vi "Sequence.Start.vi"(8 "error in":errorcluster, 10 "UserSets":T11, 11 "Data in":T1={"BeginTS"=timestamp(0 s since 1904-01-01), "EndTS"=timestamp(0 s since 1904-01-01), "State"=enum."Init", "Status.Work"=enum."-", "Status.Process"=enum."-", "Status.Home"=enum."-", "Status.Wabco"=enum."-", "Status.Client"=enum."-", "BreakReason"=enum."-", "BreakSource"=enum."-", "DoorLock"=FALSE, "Status.Prod"=[], "UserAction"={"Stop"=FALSE, "Pause"=FALSE, "Next"=FALSE}, "UserData"={"GuiMode"=enum."Process", "Test"={"IgnoreResults"=FALSE, "IgnoreImages"=FALSE, "ServiceMode"=FALSE}, "ContinueOrder"=FALSE}, "Error"={"status"=FALSE, "code"=0, "source"=""}, "Code"={"Ready"=FALSE, "DoubleOrder"=FALSE, "OrderDone"=FALSE, "AllowSingleSlot"=FALSE, "CheckDM"=FALSE, "ThresholdA"=0, "ThresholdB"=0, "Plate"=enum."Wabco", "ImgPath"=path "", "Variant"={"State"=enum."Init", "ImgPath"=path "", "WabcoPlate"="", "WabcoProduct"="", "ClientProduct"="", "ClientPlate"="", "TotalQuantity"=0, "OrderQuantity"=0, "Serial"=0, "Wabco"={"LaserJob"="", "AdditionalTxt"="037", "FactoryCode"="", "RevID"=0, "ForkID"=0, "FailuresLimit"=0, "GlobalCnt"=0, "Bank"=0, "SerialFormat"=enum."6 dig", "CoordA"={"X"=0.0, "Y"=0.0, "Angle"=0.0}, "CoordB"={"X"=0.0, "Y"=0.0, "Angle"=0.0}, "DMCconfig"=0}, "Client"={"LaserJob"="", "AdditionalTxt"="", "FactoryCode"="037", "RevID"=0, "ForkID"=0, "FailuresLimit"=0, "GlobalCnt"=0, "Bank"=0, "SerialFormat"=enum."6 dig", "CoordA"={"X"=0.0, "Y"=0.0, "Angle"=0.0}, "CoordB"={"X"=0.0, "Y"=0.0, "Angle"=0.0}, "DMCconfig"=0}}}, "Rotations"=0, "ProdIdx"=0, "ProdDone"=[], "PrintedSerials-Wabco"=[], "PrintedSerials-Client"=[], "Counters-Wabco"={"Expected"=0, "Done"=0, "OK"=0, "NOK"=0, "NOKlimit"=0, "Part"=0, "PartOK"=0}, "Counters-Client"={"Expected"=0, "Done"=0, "OK"=0, "NOK"=0, "NOKlimit"=0, "Part"=0, "PartOK"=0}}) -> (0 "error out":errorcluster, 3 "Data out":T1={"BeginTS"=timestamp(0 s since 1904-01-01), "EndTS"=timestamp(0 s since 1904-01-01), "State"=enum."Init", "Status.Work"=enum."-", "Status.Process"=enum."-", "Status.Home"=enum."-", "Status.Wabco"=enum."-", "Status.Client"=enum."-", "BreakReason"=enum."-", "BreakSource"=enum."-", "DoorLock"=FALSE, "Status.Prod"=[], "UserAction"={"Stop"=FALSE, "Pause"=FALSE, "Next"=FALSE}, "UserData"={"GuiMode"=enum."Process", "Test"={"IgnoreResults"=FALSE, "IgnoreImages"=FALSE, "ServiceMode"=FALSE}, "ContinueOrder"=FALSE}, "Error"={"status"=FALSE, "code"=0, "source"=""}, "Code"={"Ready"=FALSE, "DoubleOrder"=FALSE, "OrderDone"=FALSE, "AllowSingleSlot"=FALSE, "CheckDM"=FALSE, "ThresholdA"=0, "ThresholdB"=0, "Plate"=enum."Wabco", "ImgPath"=path "", "Variant"={"State"=enum."Init", "ImgPath"=path "", "WabcoPlate"="", "WabcoProduct"="", "ClientProduct"="", "ClientPlate"="", "TotalQuantity"=0, "OrderQuantity"=0, "Serial"=0, "Wabco"={"LaserJob"="", "AdditionalTxt"="037", "FactoryCode"="", "RevID"=0, "ForkID"=0, "FailuresLimit"=0, "GlobalCnt"=0, "Bank"=0, "SerialFormat"=enum."6 dig", "CoordA"={"X"=0.0, "Y"=0.0, "Angle"=0.0}, "CoordB"={"X"=0.0, "Y"=0.0, "Angle"=0.0}, "DMCconfig"=0}, "Client"={"LaserJob"="", "AdditionalTxt"="", "FactoryCode"="037", "RevID"=0, "ForkID"=0, "FailuresLimit"=0, "GlobalCnt"=0, "Bank"=0, "SerialFormat"=enum."6 dig", "CoordA"={"X"=0.0, "Y"=0.0, "Angle"=0.0}, "CoordB"={"X"=0.0, "Y"=0.0, "Angle"=0.0}, "DMCconfig"=0}}}, "Rotations"=0, "ProdIdx"=0, "ProdDone"=[], "PrintedSerials-Wabco"=[], "PrintedSerials-Client"=[], "Counters-Wabco"={"Expected"=0, "Done"=0, "OK"=0, "NOK"=0, "NOKlimit"=0, "Part"=0, "PartOK"=0}, "Counters-Client"={"Expected"=0, "Done"=0, "OK"=0, "NOK"=0, "NOKlimit"=0, "Part"=0, "PartOK"=0}})   [LabVIEW 2016]
uses:
  Sequence.UserData.ctl
  Sequence.MainMode.ctl
  Gui/MainGui.TestOptions.ctl
  Sequence.Data.ctl
  Sequence.State.ctl
  Sequence.Step.Status.ctl
  Sequence.Test.BreakReason.ctl
  Sequence.Test.BreakSource.ctl
  Sequence.Test.Status.ctl
  Sequence.Slot.StatusData.ctl
  Sequence.Test.Unload.Status.ctl
  Sequence.Prod.StatusData.ctl
  Sequence.UserActions.ctl
  Sequence.Code.Sets.ctl
  Sequence.PlateType.ctl
  Logger/Logger.Variant.Sets.ctl
  Station/Station.Changeover.State.vi
  Station/Station.Plate.Properties.ctl
  Sequence.Code.SerialFormat.ctl
  Drivers/V7310/LowLevel/V7310.Job.Sets.ctl
  Sequence.Counters.ctl
  tools/EventLog/EventLog.EventSource.ctl
  Sequence.SerialsFglb.Action.ctl
  Sequence.SerialsFglb.SerialData.ctl
  Station/Station.ProductSlot.ctl
  tools/Translator/Translator.Message.ctl
  Station/Station.Global.vi
  tools/EventLog/EventLog.New(array).vi
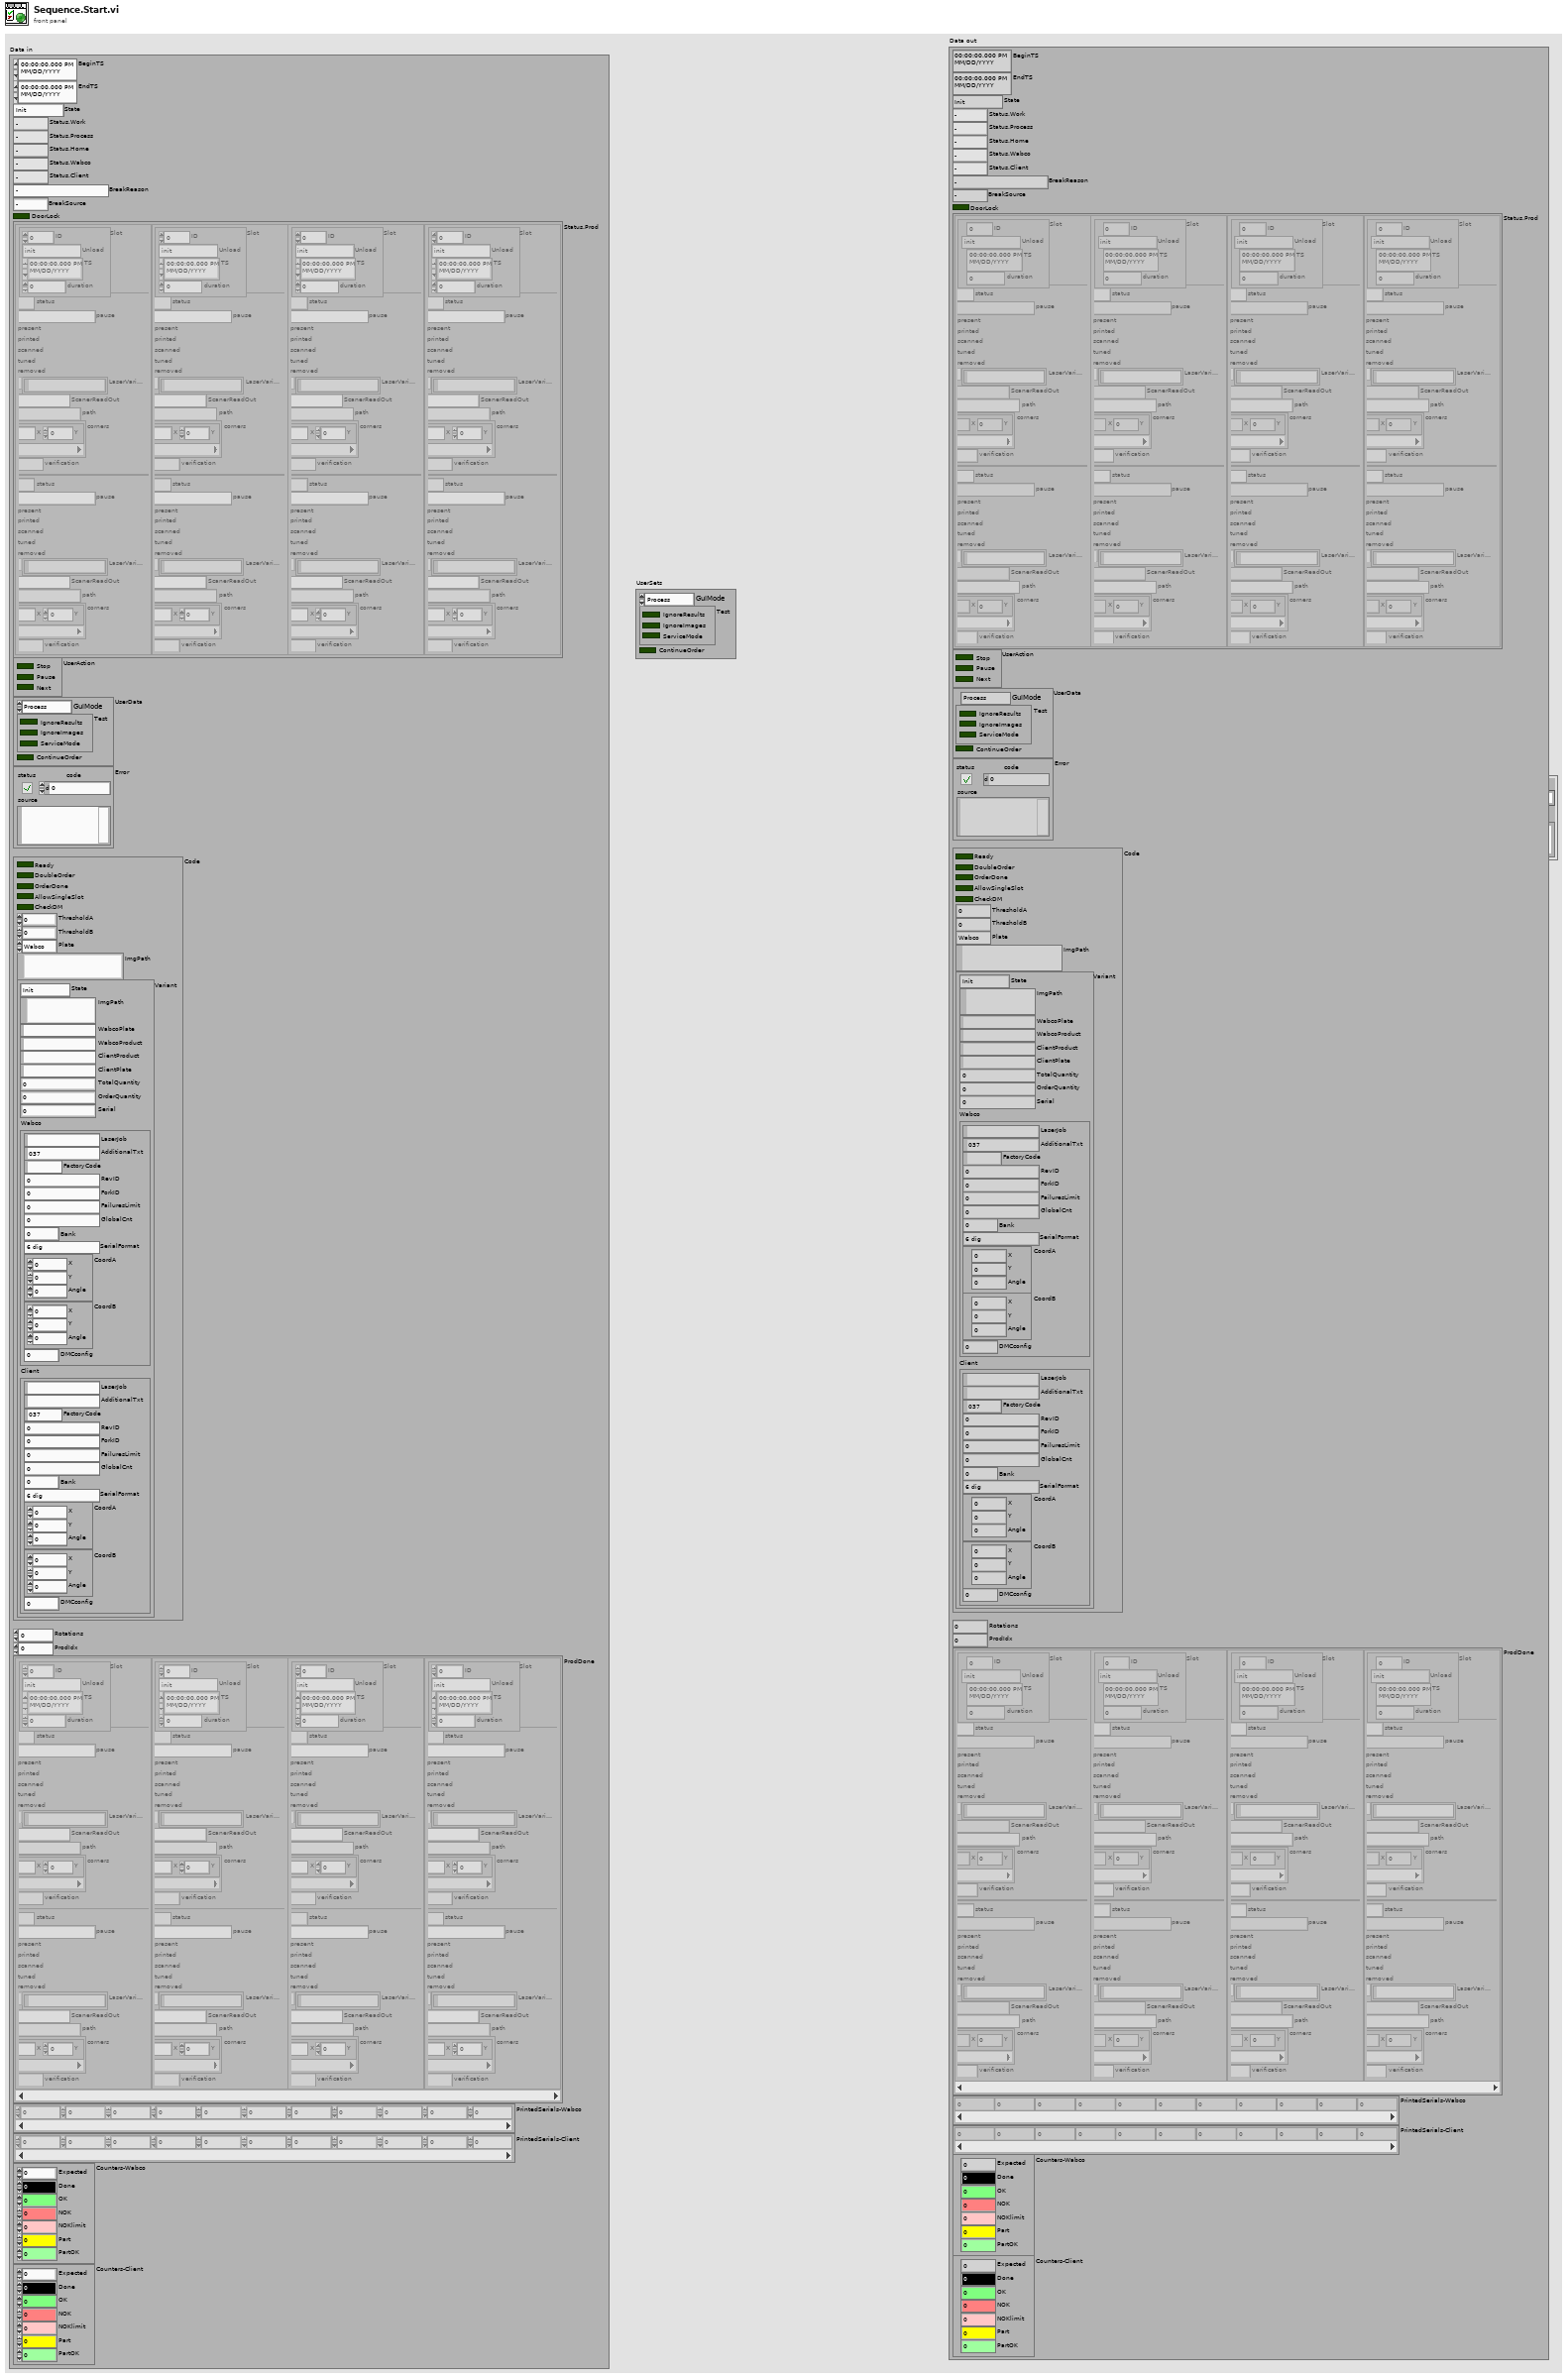
[diagram p1: front panel]
types:
  T1 = typedef "Sequence.Data.ctl" = cluster{"BeginTS":timestamp, "EndTS":timestamp, "State":T2, "Status.Work":T3, "Status.Process":T3, "Status.Home":T3, "Status.Wabco":T3, "Status.Client":T3, "BreakReason":T4, "BreakSource":T5, "DoorLock":bool, "Status.Prod":T6[], "UserAction":T10, "UserData":T11, "Error":errorcluster, "Code":T14, "Rotations":i32, "ProdIdx":i32, "ProdDone":T6[], "PrintedSerials-Wabco":i32[], "PrintedSerials-Client":i32[], "Counters-Wabco":T21, "Counters-Client":T21}
  T2 = typedef "Sequence.State.ctl" = enum16{"Init", "Idle", "Home", "Work", "Run", "Pause"}
  T3 = typedef "Sequence.Step.Status.ctl" = enum16{"-", "Pending", "Running", "Skipped", "Passed", "Failed", "Done", "Error", "Aborted", "Stopped"}
  T4 = typedef "Sequence.Test.BreakReason.ctl" = enum16{"-", "NOK container", "OK container", "Rev empty", "Rev missing", "Rev wrong", "Fork missing", "Fork wrong", "NOK limit", "Unload failure", "Single slot", "Part done", "Err: Prod move work", "Err: Prod move home", "Err: Prod lift work", "Err: Prod lift home", "Err: Prod Arm Work", "Err: Prod Arm NOK", "Err: Prod Arm OK", "Err: Prod NOK suck", "Err: Prod NOK drop", "Err: Prod OK missing", "Err: Prod OK suck", "Err: Prod OK drop"}
  T5 = typedef "Sequence.Test.BreakSource.ctl" = enum16{"-", "A", "B", "A/B"}
  T6 = typedef "Sequence.Test.Status.ctl" = cluster{"Slot":T7, "A":T9, "B":T9}
  T7 = typedef "Sequence.Slot.StatusData.ctl" = cluster{"ID":i32, "Unload":T8, "TS":timestamp, "duration":u32}
  T8 = typedef "Sequence.Test.Unload.Status.ctl" = enum16{"init", "check NOK", "check OK", "wait on NOK", "wait on OK", "wait on Unload", "done"}
  T9 = typedef "Sequence.Prod.StatusData.ctl" = cluster{"status":T3, "pause":T4, "present":bool, "printed":bool, "scanned":bool, "tuned":bool, "removed":bool, "LaserVariables":string[], "ScanerReadOut":string, "path":path, "corners":cluster{"X":i32, "Y":i32}[], "verification":u8}
  T10 = typedef "Sequence.UserActions.ctl" = cluster{"Stop":bool, "Pause":bool, "Next":bool}
  T11 = typedef "Sequence.UserData.ctl" = cluster{"GuiMode":T12, "Test":T13, "ContinueOrder":bool}
  T12 = typedef "Sequence.MainMode.ctl" = enum16{"Process", "Base", "Order", "Manual", "Logs", "Results", "Stats", "DMC Config"}
  T13 = typedef "MainGui.TestOptions.ctl" = cluster{"IgnoreResults":bool, "IgnoreImages":bool, "ServiceMode":bool}
  T14 = typedef "Sequence.Code.Sets.ctl" = cluster{"Ready":bool, "DoubleOrder":bool, "OrderDone":bool, "AllowSingleSlot":bool, "CheckDM":bool, "ThresholdA":u8, "ThresholdB":u8, "Plate":T15, "ImgPath":path, "Variant":T16}
  T15 = typedef "Sequence.PlateType.ctl" = enum16{"Wabco", "Client"}
  T16 = typedef "Logger.Variant.Sets.ctl" = cluster{"State":T17, "ImgPath":path, "WabcoPlate":string, "WabcoProduct":string, "ClientProduct":string, "ClientPlate":string, "TotalQuantity":u16, "OrderQuantity":u16, "Serial":i32, "Wabco":T18, "Client":T18}
  T17 = typedef "Station.Changeover.State.vi" = enum16{"Init", "Scaning", "NOK", "Wait for ack", "Ready"}
  T18 = typedef "Station.Plate.Properties.ctl" = cluster{"LaserJob":string, "AdditionalTxt":string, "FactoryCode":string, "RevID":u8, "ForkID":u8, "FailuresLimit":u16, "GlobalCnt":i32, "Bank":u8, "SerialFormat":T19, "CoordA":T20, "CoordB":T20, "DMCconfig":i32}
  T19 = typedef "Sequence.Code.SerialFormat.ctl" = enum8{"", "6 dig", "7 dig"}
  T20 = typedef "V7310.Job.Sets.ctl" = cluster{"X":dbl, "Y":dbl, "Angle":dbl}
  T21 = typedef "Sequence.Counters.ctl" = cluster{"Expected":u16, "Done":u16, "OK":u16, "NOK":u16, "NOKlimit":u16, "Part":u16, "PartOK":u16}
  T22 = typedef "Translator.Message.ctl" = enum16{"-", "Event confirmed", "Log out", "Log in", "Shutdown", "Cancel", "Start", "Begin time", "End time", "Duration", "Service Mode", "Ignore Results", "Serial Format", "On", "Off", "OK", "NOK", "NOK %s", "Home", "Work", "Close", "Open", "In progress...", "Missing", "Empty", "Hardware failure", "Initial", "Default", "Total", "Out of range", "Free disk space is below 1GB - contact technician", "Error %d >> %s", "Error %d >> %s >> %s", "Msg %d >> %s", "Laser msg %d %s", "Laser cmd error %s %d", "Laser cmd failed %s", "Laser cmd warning %s", "Laser disconnected", "Laser status %s", "Laser already started", "Laser job unkonwn %s", "Laser job missing %s", "Laser job select failure %s", "Unable to start laser printing (%s)", "Unable to stop laser printing (%s)", "Laser marking aborted", "Laser marking timeout", "Unable to reset Laser Interlock (%s)", "Unable to trigger Laser. Laser not ready (%s)", "Laser job '%s' coordinates not configured", "Starting %s", "Quitting %s", "Configured", "Initializing", "Quitting", "Loading", "Loaded %d results", "Loaded %d events", "Running", "Stopped", "Summary", "Laser", "Do you want to continue?", "Do you want to delete the configuration?", "The configuration is being used by an order. Unable to delete!", "Press confirm button", "Station is not based. Do you want to exit?", "Station requires changeover. Do you want to run the test?", "Test options are not set as default. Do you want to continue?", "Formatting of WabcoNo is disabled. Do you want to continue?", "Product not detected. Do you want to continue?", "Product scan failed. Do you want to continue?", "Calibration", "Log out?", "System", "All", "IDLE", "Translating...%s", "Not found", "Alarm %s", "Run", "Skip", "Abort", "Repeat", "Please wait...", "Database disconnected", "Database disconnected - changeover disabled!", "Login to database successful", "Login to database failed: %d; %s", "Unable to check the product status of reference %d - database disconnected", "Unable to set the product status of reference %d - database disconnected", "Variant file backup %s", "Read variant (%s)", "Result", "Station armed!", "Station requires changeover!", "Select reference number...", "EMERGENCY BUTTON - press Control button", "EMERGENCY DOOR - press Control button", "Resetting Emergency...", "Unable to reset safety circuit - Emergency Button pressed", "Unable to reset safety circuit - Emergency Side Door open", "Station not based", "Station based", "Station not empty", "Station basing...", "No order", "Press Start to begin new order", "Scanning new order", "Order NOK. Correct or scan again", "Order OK. Press Accept", "Order ready", "Revolver incorrect", "Fork incorrect", "Revolver missing", "Revolver empty", "Container missing", "Offline results", "Offline statistics", "Updating statistics %.1f %%", "DMC Configurator", "Door open", "Close the front door", "Press start button", "Done. Open the front door", "Running...", "Running...%.1f %%", "Pause %s", "Pause %s. NOK container missing", "Pause %s. OK container missing", "Pause %s. Revolver empty", "Pause %s. Revolver missing", "Pause %s. Revolver incorrect", "Pause %s. Fork missing", "Pause %s. Fork incorrect", "Pause %s. Too many failures", "Pause %s. Unloading failure", "Pause %s. One slot is not working", "Pause %s. Part order is done. Empty OK container", "Pause %s. Unable to move product to slot", "Pause %s. Unable to move back product pusher", "Pause %s. Unable to lift product", "Pause %s. Unable to move back product lifter", "Pause %s. Unable to move product arm to Work", "Pause %s. Unable to move product arm to NOK", "Pause %s. Unable to move product arm to OK", "Pause %s. Unable to unsuck the NOK product", "Pause %s. Unable to drop the NOK product", "Pause %s. Product OK missing", "Pause %s. Unable to unsuck the OK product", "Pause %s. Unable to drop the OK product", "Stopping...", "File '%s' is missing", "File '%s' is broken", "File '%s' is running", "Log file started (%s)", "Log file ended (%s)", "Log file stopped (%s)", "Log file ignored (%s)", "Log file exported (%s)", "Log file export failed (%s)", "Wrong serial number in log file", "Wrong reference number in log file", "Test steps are missing", "%s = %.3f", "Process param '%s' not found in DB", "Process param '%s' wrong order", "Process param '%s' value %.3f out of limits (%.3f; %.3f)", "Step%d param '%s' not found in DB", "Step%d param '%s' wrong order", "Step%d param '%s' value %.3f out of limits (%.3f; %.3f)", "Step%d EV '%s' not found in DB", "Step%d EV '%s' wrong order", "\"%s\" not found in DB", "\"%s\" wrong order", "\"%s\" value %.3f out of limits (%.3f; %.3f)", "\"%s\" not found in software", "Process init (%s)", "Process started", "Process restarted", "Process run", "Process done", "Process done - remove OK container", "Process aborted", "Process aborted at work", "Process aborted at home", "Process error", "Process error at home", "Process error at work", "Process close", "Process pause", "Process continue", "Process door open", "Process door close", "Process pause at slot %s due to %s", "Select plate from the order to process", "Do you want to start the process?", "Do you want to continue the process?", "There is unfinished order. Do you want to put the new order?", "Product %s %d OK", "Product %s %d NOK", "Unable to unload the slot %s. Product missing in the slot", "Unable to unload the slot %s. Product already in the arm", "Unable to accept the product as OK. Product missing in slot %s", "Unable to accept the product as OK. Product could not drop into the container at slot %s", "Unable to accept the product as NOK. Product could not drop into the container at slot %s", "Scan failed. Error %s", "Scan failed. Scanner disconnected", "Scan failed. Wrong Wabco number %d, limit (%d,%d)", "Scan failed. Wrong serial number %d, limit (%d,%d)", "Scan failed. Wrong date %d, limit (%d,%d)", "Scan failed. Wrong product wabco number %d (expected %d)", "Scan failed. Wrong product serial number %d (expected > 0)", "Scan OK %s", "Scan failed. Unable to determine table position (%s)", "Scan failed. Timeout", "Tune failed. Scanner disconnected", "Tune failed. Timeout", "%s = %d", "%s = %d->%d", "Unable to set %s = %.2f - Air Pressure Inside off", "Unable to set digital output '%s' = %d", "Unable to activate air pressure inside - timeout", "Unable to activate air pressure inside - aborted", "Unable to switch on Air Main Valve - Air Pressure Inlet off", "Unable to switch on Air Main Valve - Door open", "Unable to switch off Air Main Valve - timeout", "Unable to switch off Air Main Valve - aborted", "Unable to rotate Table - timeout", "Unable to rotate Table - aborted", "Unable to rotate Table - Product Move not in Home position", "Unable to rotate Table - Air Pressure Inside off", "Unable to rotate Table - Product Lift A not in Home position", "Unable to rotate Table - Product Lift B not in Home position", "Unable to rotate Table - unlock before movement timeout", "Unable to rotate Table - lock after movement timeout", "Unable to move Table Lock to %s position - timeout", "Unable to move Table Lock to %s position - aborted", "Unable to move Table Lock to %s position - Air Pressure Inside off", "Unable to move Table Lock to %s position - Table not in position", "Unable to move Product Lift A to %s position - timeout", "Unable to move Product Lift B to %s position - timeout", "Unable to move Product Lift A to %s position - aborted", "Unable to move Product Lift B to %s position - aborted", "Unable to move Product Lift A to %s position - Air Pressure Inside off", "Unable to move Product Lift B to %s position - Air Pressure Inside off", "Unable to move Product Lift A to %s position - Table not locked", "Unable to move Product Lift B to %s position - Table not locked", "Unable to move Product Lift A to %s position - Product Arm not in Work position", "Unable to move Product Lift B to %s position - Product Arm not in Work position", "Unable to set Product Suction Gripper %s to %s - timeout", "Unable to set Product Suction Gripper %s to %s - aborted", "Unable to set Product Suction Gripper %s to %s - Air Pressure Inside off", "Unable to set Product Suction Gripper %s to %s - Table slot unkown", "Unable to move Product Arm to %s position - timeout", "Unable to move Product Arm to %s position - aborted", "Unable to move Product Arm to %s position - Air Pressure Inside off", "Unable to move Product Arm to %s position - Product Lift A not in Home position", "Unable to move Product Arm to %s position - Product Lift B not in Home position", "Unable to move Product to %s position - timeout", "Unable to move Product to %s position - aborted", "Unable to move Product to %s position - Air Pressure Inside off", "Unable to move Product to %s position - Table not in position"}
  T23 = typedef "Sequence.SerialsFglb.SerialData.ctl" = cluster{"TS":timestamp, "Slot":T24, "Serial":i32, "Global":bool}
  T24 = typedef "Station.ProductSlot.ctl" = enum8{"A", "B"}
  T25 = typedef "Sequence.SerialsFglb.Action.ctl" = enum16{"init", "get", "get next", "pass", "fail", "confirm", "clean"}
  T26 = typedef "EventLog.EventSource.ctl" = enum16{"All", "Gui", "Ref", "File", "Arch", "Seq", "CPX", "DB", "Laser", "Scan.P", "Scan.O"}
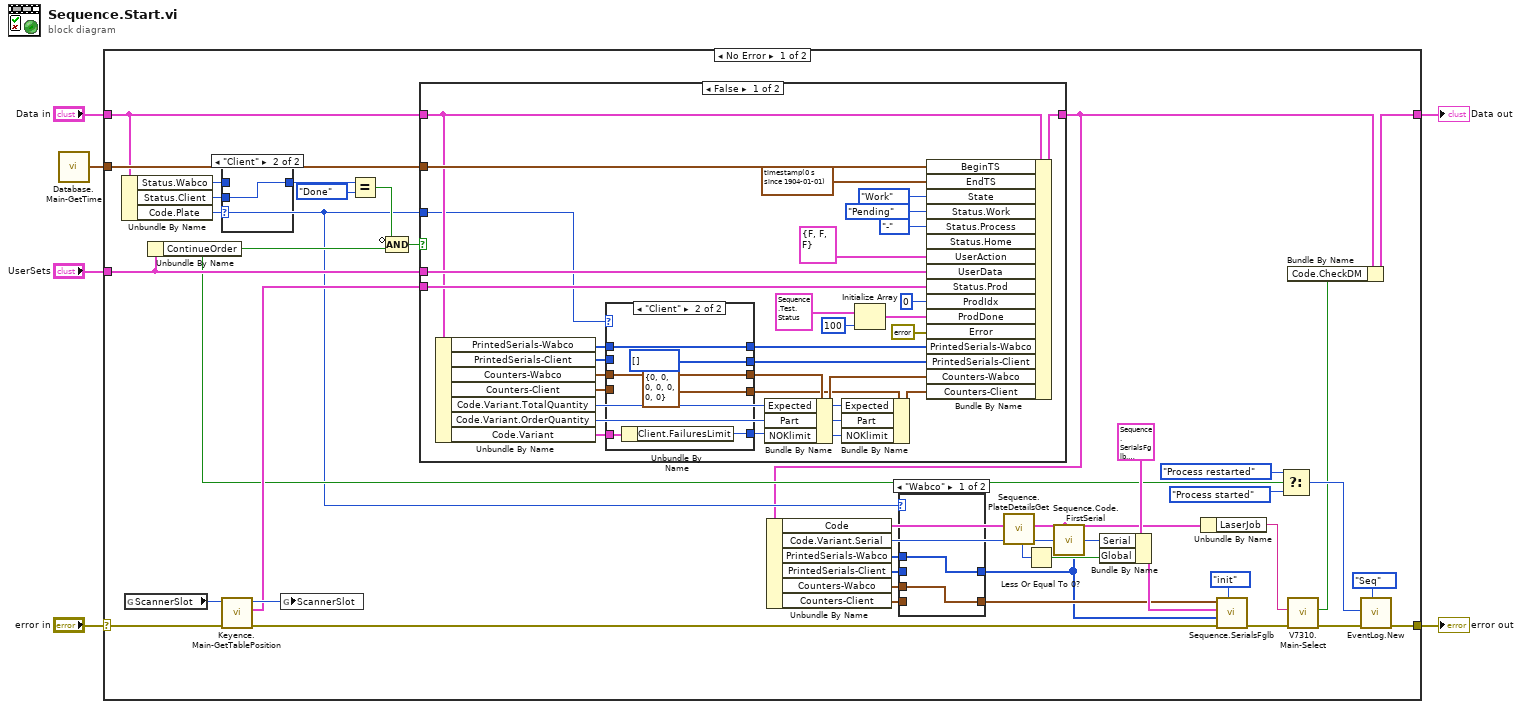
[diagram p0: block diagram]
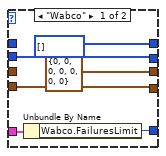
[diagram p4: hidden frame]
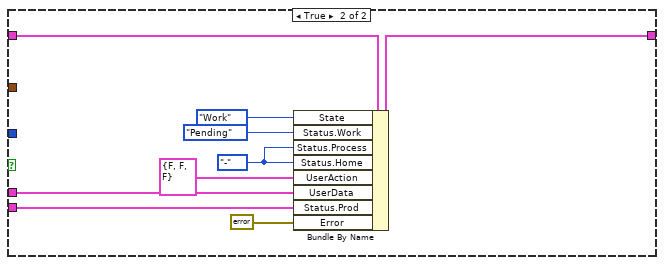
[diagram p5: hidden frame]
diagram:
  n1 = call "Database.Main-GetTime.vi"() -> ("TS"=w1:timestamp)  [unwired: 1 in]
  n2 = case shown="No Error" "error in" {
    selector: "error in" -> [w34 w105]
    tunnel: "UserSets" -> [w45 _]
    tunnel: [w47 w105] -> w5
    tunnel: "Data in" -> [w27 w106]
    tunnel: w1 -> [w46 _]
    tunnel: [w10 w106] -> w2
    frame No Error {
      n3 = Unbundle By Name(w27) -> ("Status.Wabco"=w30:T3, "Status.Client"=w31:T3, "Code.Plate"=w20:T15)
      n4 = global read "Station.Global.vi" "ScannerSlot"() -> (w38:i32)
      n5 = Unbundle By Name(w45) -> ("ContinueOrder"=w24:bool)
      n6 = case shown="\"Client\"" w20 {
        tunnel: [w52 w53] -> w29
        tunnel: w31 -> [_ w53]
        tunnel: w30 -> [w52 _]
        frame "Wabco" {
        }
        frame "Client" {
        }
      }
      n7 = call "Keyence.Main-GetTablePosition.vi"("error in (no error)"=w34, "ScannerSlot in"=w38) -> ("error out"=w35:errorcluster, "TestStatus"=w36:T6[], "ScannerSlot out"=w37:i32)  [unwired: 7 in]
      n8 = global write "Station.Global.vi" "ScannerSlot"(w37) -> ()
      n9 = Equal?(x=w29, y=Sequence.Step.Status."Done") -> (x = y?=w25:bool)
      n10 = Compound Arithmetic op=AND(invert w25, w24) -> (w26:bool)
      n11 = case shown="False" w26 {
        tunnel: w27 -> [w69 w103]
        tunnel: w46 -> [w71 _]
        tunnel: [w83 w104] -> w9
        tunnel: w45 -> [w74 w99]
        tunnel: w36 -> [w72 w96]
        tunnel: w20 -> [w68 _]
        frame False {
          w70 = Sequence.Step.Status."-" ("Status.Home")
          n12 = Unbundle By Name(w69) -> ("PrintedSerials-Wabco"=w67:i32[], "PrintedSerials-Client"=w66:i32[], "Counters-Wabco"=w63:T21, "Counters-Client"=w62:T21, "Code.Variant.TotalQuantity"=w57:u16, "Code.Variant.OrderQuantity"=w56:u16, "Code.Variant"=w55:T16)
          n13 = case shown="\"Client\"" w68 {
            tunnel: [i32[] [] ("PrintedSerials") w95] -> w65
            tunnel: w67 -> [_ w95]
            tunnel: w66 -> [w88 _]
            tunnel: [w88 i32[] [] ("PrintedSerials")] -> w64
            tunnel: w63 -> [_ w93]
            tunnel: w62 -> [w87 _]
            tunnel: [T21 {"Expected"=0, "Done"=0, "OK"=0, "NOK"=0, "NOKlimit"=0, "Part"=0, "PartOK"=0} ("Counters") w93] -> w61
            tunnel: [w87 T21 {"Expected"=0, "Done"=0, "OK"=0, "NOK"=0, "NOKlimit"=0, "Part"=0, "PartOK"=0} ("Counters")] -> w59
            tunnel: w55 -> [w85 w91]
            tunnel: [w84 w90] -> w54
            frame "Wabco" {
              n14 = Unbundle By Name(w85) -> ("Wabco.FailuresLimit"=w84:u16)
            }
            frame "Client" {
              n15 = Unbundle By Name(w91) -> ("Client.FailuresLimit"=w90:u16)
            }
          }
          n16 = Bundle By Name(cluster=w61, "Expected"=w57, "Part"=w56, "NOKlimit"=w54) -> (w60:T21)
          n17 = Bundle By Name(cluster=w59, "Expected"=w57, "Part"=w56, "NOKlimit"=w54) -> (w58:T21)
          n18 = Initialize Array(T6 {"Slot"={"ID"=0, "Unload"=enum."init", "TS"=timestamp(0 s since 1904-01-01), "duration"=0}, "A"={"status"=enum."-", "pause"=enum."-", "present"=FALSE, "printed"=FALSE, "scanned"=FALSE, "tuned"=FALSE, "removed"=FALSE, "LaserVariables"=[], "ScanerReadOut"="", "path"=path "", "corners"=[], "verification"=0}, "B"={"status"=enum."-", "pause"=enum."-", "present"=FALSE, "printed"=FALSE, "scanned"=FALSE, "tuned"=FALSE, "removed"=FALSE, "LaserVariables"=[], "ScanerReadOut"="", "path"=path "", "corners"=[], "verification"=0}} ("Data in"), 100 ("dimension size")) -> (w79:T6[])
          n19 = Bundle By Name(cluster=w69, "BeginTS"=w71, "EndTS"=timestamp(0 s since 1904-01-01), "State"=Sequence.State."Work", "Status.Work"=Sequence.Step.Status."Pending" ("Status.Home"), "Status.Process"=w70, "Status.Home"=w70, "UserAction"=T10 {"Stop"=FALSE, "Pause"=FALSE, "Next"=FALSE}, "UserData"=w74, "Status.Prod"=w72, "ProdIdx"=0, "ProdDone"=w79, "Error"=errorcluster {"status"=FALSE, "code"=0, "source"=""}, "PrintedSerials-Wabco"=w65, "PrintedSerials-Client"=w64, "Counters-Wabco"=w60, "Counters-Client"=w58) -> (w83:T1)
        }
        frame True {
          w97 = Sequence.Step.Status."-" ("Status.Home")
          n20 = Bundle By Name(cluster=w103, "State"=Sequence.State."Work", "Status.Work"=Sequence.Step.Status."Pending" ("Status.Home"), "Status.Process"=w97, "Status.Home"=w97, "UserAction"=T10 {"Stop"=FALSE, "Pause"=FALSE, "Next"=FALSE}, "UserData"=w99, "Status.Prod"=w96, "Error"=errorcluster {"status"=FALSE, "code"=0, "source"=""}) -> (w104:T1)
        }
      }
      n21 = Unbundle By Name(w9) -> ("Code"=w33:T14, "Code.Variant.Serial"=w15:i32, "PrintedSerials-Wabco"=w19:i32[], "PrintedSerials-Client"=w18:i32[], "Counters-Wabco"=w17:T21, "Counters-Client"=w16:T21)
      n22 = case shown="\"Wabco\"" w20 {
        tunnel: w19 -> [w49 _]
        tunnel: w18 -> [_ w51]
        tunnel: [w49 w51] -> w7
        tunnel: w17 -> [w48 _]
        tunnel: w16 -> [_ w50]
        tunnel: [w48 w50] -> w13
        frame "Wabco" {
        }
        frame "Client" {
        }
      }
      n23 = call "Sequence.PlateDetailsGet.vi"("Code in"=w33) -> ("PlateDetails"=w32:T18)  [unwired: 9 in, 1 out]
      n24 = Less Or Equal To 0?(x=w15) -> (x <= 0?=w14:bool)
      n25 = call "Sequence.Code.FirstSerial.vi"("Serial in"=w15, "Code"=w32, "Printed serials"=w7) -> ("Serial out"=w40:i32)
      n26 = Bundle By Name(cluster=T23 {"TS"=timestamp(0 s since 1904-01-01), "Slot"=enum."A", "Serial"=0, "Global"=FALSE} ("SerialData"), "Serial"=w40, "Global"=w14) -> (w39:T23)
      n27 = Unbundle By Name(w32) -> ("LaserJob"=w41:string)
      n28 = call "Sequence.SerialsFglb.vi"("Action (get)"=Sequence.SerialsFglb.Action."init", "error in"=w35, "Printed serials in"=w7, "Serial data in"=w39, "Counters in"=w13) -> ("error out"=w12:errorcluster)  [unwired: 2 in, 4 out]
      n29 = Select(t=Translator.Message."Process restarted" ("msg"), s=w24, f=Translator.Message."Process started" ("msg")) -> (s? t:f=w21:T22)
      n30 = call "V7310.Main-Select.vi"("error in"=w12, "Name"=w41) -> ("error out"=w11:errorcluster, "CheckDM"=w8:bool)  [unwired: 8 in]
      n31 = Bundle By Name(cluster=w9, "Code.CheckDM"=w8) -> (w10:T1)
      n32 = call-poly "EventLog.New.vi"("Source (All)"=EventLog.EventSource."Seq", "error in (no error)"=w11, "Message (-)"=w21) -> ("error out"=w47:errorcluster)  [unwired: 7 in, 1 out]
    }
    frame Error {
    }
  }
  "error out" <- w5
  "Data out" <- w2
